vi "NameJSONtoPersonnelJSON.vi"(11 "Name JSON":string) -> (3 "Personnel JSON":string)   [LabVIEW 2015]
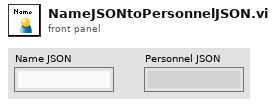
[diagram p1: front panel]
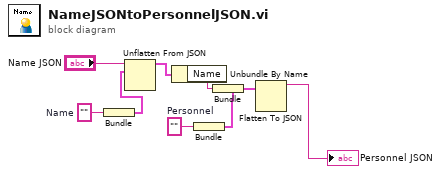
[diagram p0: block diagram]
diagram:
  w5 = ""  # Personnel
  w1 = ""  # Name
  n1 = Bundle("Name"=w1) -> (w3:cluster{"Name":string})  [unwired: 1 in]
  n2 = Unflatten From JSON(JSON string="Name JSON", type and defaults=w3) -> (value=w4:cluster{"Name":string})  [unwired: 5 in, 1 out]
  n3 = Unbundle By Name(w4) -> ("Name"=w6:string)
  n4 = Bundle("Personnel"=w5) -> (w7:cluster{"Personnel":string})  [unwired: 1 in]
  n5 = Bundle(cluster=w7, "Personnel"=w6) -> (w8:cluster{"Personnel":string})
  n6 = Flatten To JSON(anything=w8) -> (JSON string=→"Personnel JSON":string)  [unwired: 2 in, 1 out]
